vi "Tracking IOL.vi"(5 "Trajectory Cluster":T3, 6 "OCT Z PID Gains":cluster{"Kp":dbl, "Kd":dbl, "Ki":dbl}={"Kp"=0.0003, "Kd"=0.0001, "Ki"=0.01}, 7 "Eye Model Cluster":T2={"X Grid"=[], "Y Grid"=[], "Za_true Surf"=[], "Iris Center"=[], "Zp_true Surf"=[], "Pinv"=[[1.0, 0.0], [0.0, 1.0]], "za_true"=5.0, "za_work"=1.0, "zp_work"=-1.0, "zp_true"=-5.0}, 8 "error in":errorcluster, 9 "OCT Prev Posit":dbl, 10 "Resume Index":i32, 11 "FPGA VI Reference In":refnum<k20>) -> (0 "error out":errorcluster, 1 "OCT Last Posit":dbl, 2 "Leave Index":i32, 3 "FPGA VI Reference Out":refnum<k20>)   [LabVIEW 2016]
uses:
  Subsystems/Global Variables.vi
  <vilib>/Platform/TimedLoop/XDataNode/wakeup.ctl
  <vilib>/Platform/TimedLoop/XDataNode/XDNodeRunTimeDep.lvlib
  <vilib>/Platform/TimedLoop/XDataNode/nitl_modes.ctl
  <vilib>/Platform/TimedLoop/XDataNode/timing_clust.ctl
  <vilib>/platform/TimedLoop/XDataNode/XDataNode.xnode
  Library/KevinLibraryAll/labview/KevLib01.lvlib
  <vilib>/Analysis/Matrix/Datatypes/RealMatrix.ctl
  <vilib>/Analysis/Matrix/NI_Matrix.lvlib
panel:
  out "In Servo Loop":bool
  out "PC z Displacement":dbl
  out "Speed Schedule":dbl
  out "joint limits":dbl[][](array[numeric])=[[-10.0, 35.0], [-35.0, 35.0], [0.1, 10.0], [-40.0, 40.0]]
  out "Vac Extremum":dbl[](array[numeric])
  out "z Dist Thld":dbl[](array[numeric])
  out "z Rot Axis":dbl
  out "Deform Array":dbl[](array[numeric])=[1.0, 1.0, 1.0, 0.0, 0.0, 0.0, 0.0, 0.0, 0.0]
  out "Speed Override":u16(ring)=3 items=["4x", "3x", "2x", "1x", "0.5x", "0.2x", "0.1x", "PAUSE"]
  out "Loading Finished":bool
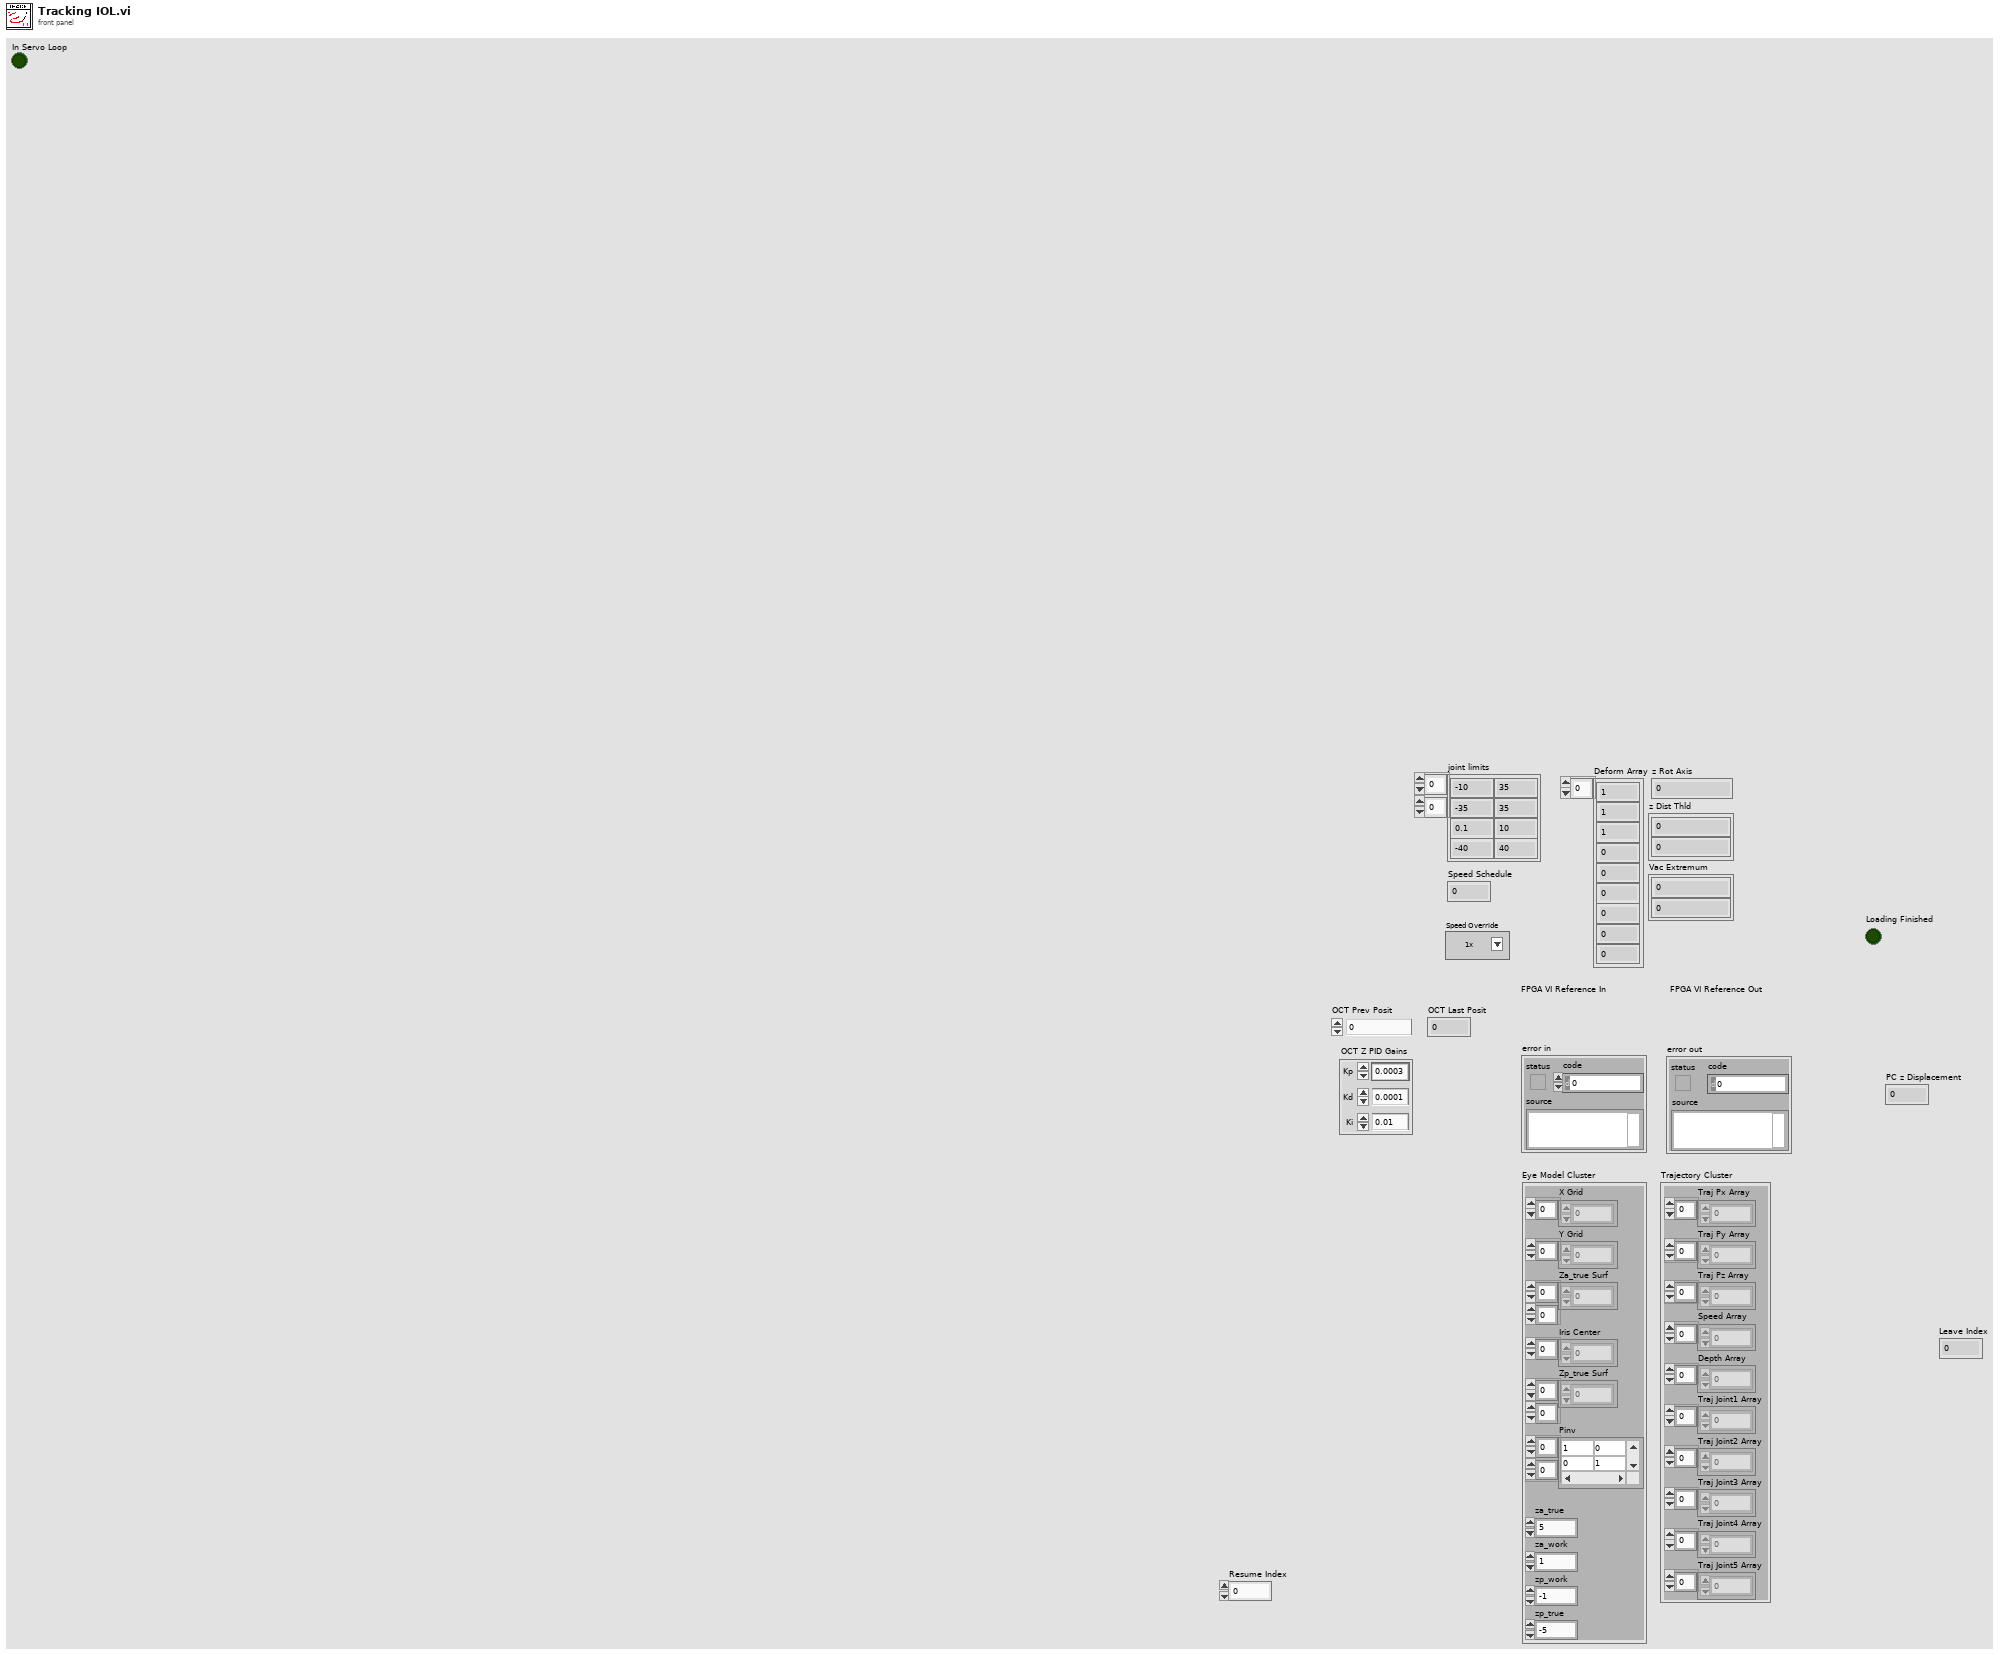
[diagram p1: front panel]
types:
  T1 = typedef "NI_Matrix.lvlib/RealMatrix.ctl" = dbl[][]
  T2 = cluster{"X Grid":dbl[], "Y Grid":dbl[], "Za_true Surf":dbl[][], "Iris Center":dbl[], "Zp_true Surf":dbl[][], "Pinv":T1, "za_true":dbl, "za_work":dbl, "zp_work":dbl, "zp_true":dbl}
  T3 = cluster{"Traj Px Array":dbl[], "Traj Py Array":dbl[], "Traj Pz Array":dbl[], "Speed Array":dbl[], "Depth Array":dbl[], "Traj Joint1 Array":dbl[], "Traj Joint2 Array":dbl[], "Traj Joint3 Array":dbl[], "Traj Joint4 Array":dbl[], "Traj Joint5 Array":dbl[]}
  T4 = typedef "XDNodeRunTimeDep.lvlib/timing_clust.ctl" = cluster{"Expected End [f-1]":u64, "Actual End [f-1]":u64, "Finished Late? [f-1]":bool, "Expected End [i-1]":u64, "Actual End [i-1]":u64, "Finished Late? [i-1]":bool, "Expected Start [i]":u64, "Actual Start [i]":u64, "Expected Start [f]":u64, "Actual Start [f]":u64, "Source Name":string, "Structure Name":string, "Period":i64, "Deadline":i64, "Offset":i64, "Start":i64, "Priority":i32, "Timeout":i32, "Mode":T5, "Wakeup Reason":T6, "Error":errorcluster, "Source Type":string, "Secondary Source Type":string, "Global End Time":u64, "Global Start Time":u64, "Frame Duration":u64, "Iteration Duration":u64, "Assigned CPU":i32, "I/O Scan Engine Mode":u32}
  T5 = typedef "XDNodeRunTimeDep.lvlib/nitl_modes.ctl" = enum32{"No Change", "Process missed periods, maintain original phase", "Discard missed periods, maintain original phase", "Process missed periods, ignore original phase", "Discard missed periods, ignore original phase"}
  T6 = typedef "XDNodeRunTimeDep.lvlib/wakeup.ctl" = enum32{"Normal", "Aborted", "Asynchronous wakeup", "Timing source error", "Timed loop error", "Timeout"}
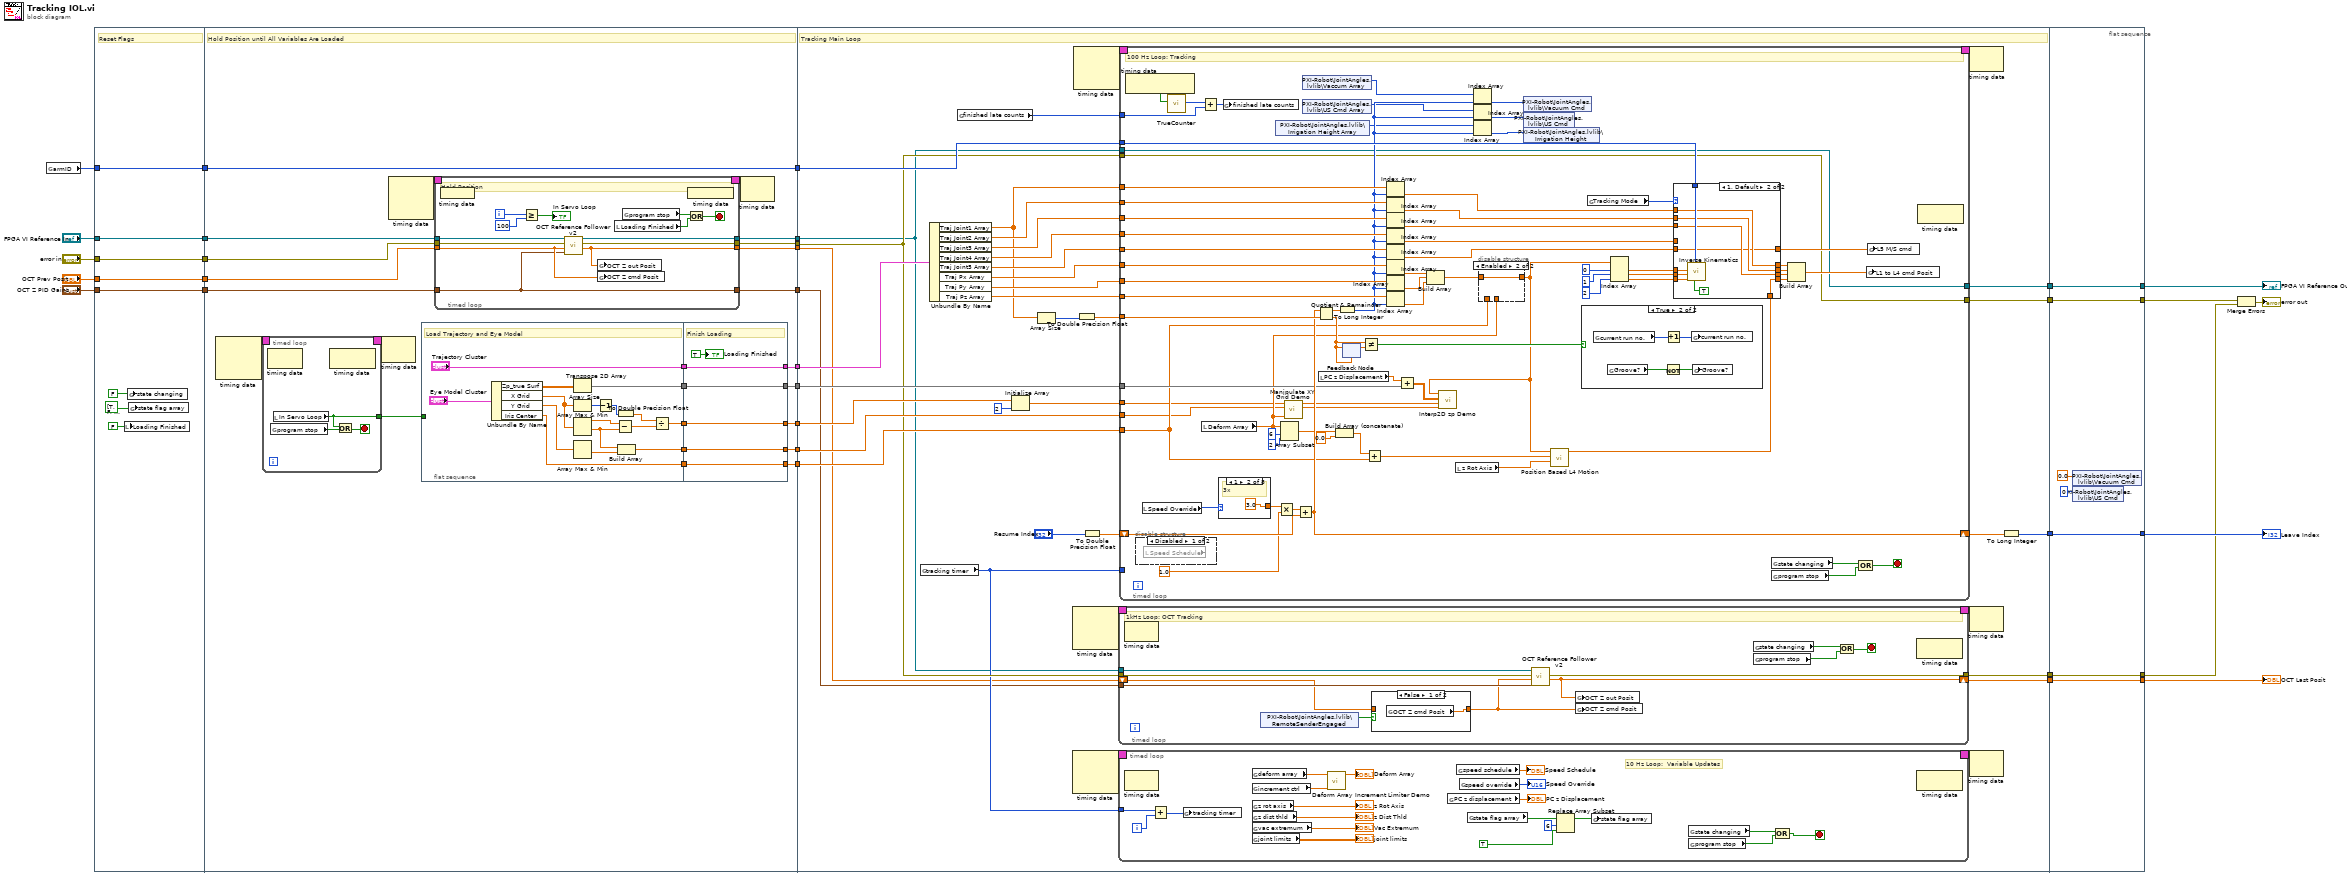
[diagram p0: block diagram]
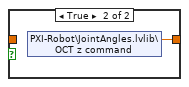
[diagram p2: hidden frame]
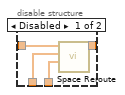
[diagram p5: hidden frame]
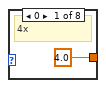
[diagram p6: hidden frame]
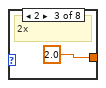
[diagram p7: hidden frame]
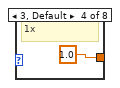
[diagram p8: hidden frame]
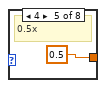
[diagram p9: hidden frame]
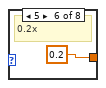
[diagram p10: hidden frame]
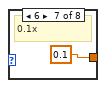
[diagram p11: hidden frame]
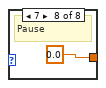
[diagram p12: hidden frame]
diagram:
  n1 = global read "Global Variables.vi" "armID"() -> (w13:i32)
  n2 = flat-sequence {
    tunnel: [w37] -> w31
    tunnel: "FPGA VI Reference In" -> [w37]
    tunnel: "error in" -> [w36]
    tunnel: [w36] -> w28
    tunnel: w13 -> [w35]
    tunnel: [w35] -> w15
    tunnel: [w33] -> w12
    tunnel: "OCT Prev Posit" -> [w33]
    tunnel: [w32] -> w10
    tunnel: "OCT Z PID Gains" -> [w32]
    tunnel: w31 -> [w50]
    tunnel: w28 -> [w49]
    tunnel: [w45] -> w27
    tunnel: [w63] -> w23
    tunnel: [w62] -> w22
    tunnel: [w61] -> w21
    tunnel: [w60] -> w19
    tunnel: [w59] -> w18
    tunnel: [w53] -> w17
    tunnel: w15 -> [w53]
    tunnel: [w46] -> w14
    tunnel: w12 -> [w48]
    tunnel: w10 -> [w47]
    tunnel: [w41] -> w8
    tunnel: [w40] -> w7
    tunnel: w27 -> [w125]
    tunnel: w23 -> [w139]
    tunnel: w22 -> [w131]
    tunnel: w21 -> [w140]
    tunnel: w19 -> [w132]
    tunnel: w18 -> [w133]
    tunnel: w17 -> [w128]
    tunnel: w14 -> [w122]
    tunnel: w8 -> [w121]
    tunnel: w7 -> [w120]
    tunnel: [w144] -> w5
    tunnel: [w143] -> w4
    tunnel: [w136] -> w3
    tunnel: [w124] -> w2
    tunnel: [w119] -> w1
    tunnel: [w304] -> w6
    tunnel: [w305] -> w16
    tunnel: [w306] -> w20
    tunnel: [w307] -> w24
    tunnel: [w308] -> w25
    tunnel: w5 -> [w308]
    tunnel: w4 -> [w307]
    tunnel: w3 -> [w306]
    tunnel: w2 -> [w305]
    tunnel: w1 -> [w304]
    frame #0 {
      # "Reset Flags"
      n3 = local write "Loading Finished"(FALSE ("Loading Finished")) -> ()
      n4 = global write "Global Variables.vi" "state changing"(FALSE ("state changing")) -> ()
      n5 = global write "Global Variables.vi" "state flag array"(bool[] [TRUE, FALSE, FALSE, FALSE, FALSE, FALSE, FALSE, FALSE, FALSE] ("state flag array")) -> ()
    }
    frame #1 {
      # "Hold Position until All Variables Are Loaded"
      n6 = node-c288() -> (w44:T4)  [unwired: 3 in]
      n7 = timed-loop {
        timing: w44 -> [_]
        timing-out: [_] -> w43
        tunnel: [w64] -> w42
        stop <- w66 stop-if-true
        n8 = node-c288() -> ()  [unwired: 1 in, 1 out]
        n9 = global read "Global Variables.vi" "program stop"() -> (w65:bool)
        n10 = local read "In Servo Loop"() -> (w64:bool)
        n11 = node-c288() -> ()  [unwired: 1 in, 1 out]
        n12 = Or(x=w64, y=w65) -> (x .or. y?=w66:bool)
      }
      n13 = node-c288(w43) -> ()  [unwired: 1 out]
      n14 = node-c288() -> (w52:T4)  [unwired: 3 in]
      n15 = flat-sequence {
        tunnel: [w90] -> w58
        tunnel: [w103] -> w57
        tunnel: [w102] -> w56
        tunnel: [w89] -> w55
        tunnel: ["Trajectory Cluster"] -> w54
        tunnel: w42 -> [_]
        tunnel: [w107] -> w61
        tunnel: [w108] -> w62
        tunnel: [w109] -> w63
        tunnel: w58 -> [w109]
        tunnel: w57 -> [w108]
        tunnel: w56 -> [w107]
        tunnel: w55 -> [w105]
        tunnel: [w105] -> w60
        tunnel: [w104] -> w59
        tunnel: w54 -> [w104]
        frame #0 {
          # "Load Trajectory and Eye Model"
          n16 = Unbundle By Name("Eye Model Cluster") -> ("Zp_true Surf"=w91:dbl[][], "X Grid"=w92:dbl[], "Y Grid"=w101:dbl[], "Iris Center"=w89:dbl[])
          n17 = Transpose 2D Array(2D array=w91) -> (transposed array=w90:dbl[][])
          n18 = Array Size(array=w92) -> (size(s)=w100:i32)
          n19 = Array Max & Min(array=w92) -> (max value=w98:dbl, min value=w99:dbl)  [unwired: 2 out]
          n20 = Array Max & Min(array=w101) -> (min value=w97:dbl)  [unwired: 3 out]
          n21 = Decrement(x=w100) -> (x-1=w95:i32)
          n22 = Subtract(x=w98, y=w99) -> (x-y=w94:dbl)
          n23 = To Double Precision Float(number=w95) -> (double precision float=w96:dbl)
          n24 = Build Array(w99, w97) -> (w102:dbl[])
          n25 = Divide(x=w96, y=w94) -> (x/y=w103:dbl)
        }
        frame #1 {
          # "Finish Loading"
          "Loading Finished" <- TRUE ("Loading Finished")
        }
      }
      n26 = timed-loop {
        timing: w52 -> [_]
        timing-out: [_] -> w51
        tunnel: [w74] -> w40
        tunnel: [w71] -> w46
        tunnel: [w75] -> w45
        tunnel: w50 -> [w77]
        tunnel: w49 -> [w76]
        tunnel: w47 -> [w72]
        tunnel: w48 -> [w73]
        tunnel: [w72] -> w41
        i -> [w80]
        stop <- w83 stop-if-true
        # "Hold Position"
        n27 = node-c288 ("Output Node")() -> ()  [unwired: 1 in]
        n28 = Greater Or Equal?(x=w80, y=100) -> (x >= y?=→"In Servo Loop":bool)
        n29 = call "OCT Reference Follower v2.vi"("OCT Z PID Gains"=w72, "OCT  Z cmd Posit [mm]"=w73, "error in"=w76, "FPGA VI Reference In"=w77) -> ("OCT  Z out Posit [mm]"=w74:dbl, "error out"=w75:errorcluster, "FPGA VI Reference Out"=w71:refnum<k20>)  [unwired: 5 in]
        n30 = global write "Global Variables.vi" "OCT Z out Posit"(w74) -> ()
        n31 = global write "Global Variables.vi" "OCT Z cmd Posit"(w73) -> ()
        n32 = local read "Loading Finished"() -> (w82:bool)
        n33 = global read "Global Variables.vi" "program stop"() -> (w81:bool)
        n34 = Or(x=w81, y=w82) -> (x .or. y?=w83:bool)
        n35 = node-c288() -> ()  [unwired: 1 out]
      }
      n36 = node-c288(w51) -> ()  [unwired: 1 out]
    }
    frame #2 {
      # "Tracking Main Loop"
      n37 = global read "Global Variables.vi" "tracking timer"() -> (w123:i32)
      n38 = Unbundle By Name(w133) -> ("Traj Joint1 Array"=w112:dbl[], "Traj Joint2 Array"=w118:dbl[], "Traj Joint3 Array"=w117:dbl[], "Traj Joint4 Array"=w116:dbl[], "Traj Joint5 Array"=w113:dbl[], "Traj Px Array"=w115:dbl[], "Traj Py Array"=w138:dbl[], "Traj Pz Array"=w134:dbl[])
      n39 = global read "Global Variables.vi" "finished late counts"() -> (w145:u16)
      n40 = Initialize Array(w131, 2 ("dimension size")) -> (w129:dbl[])
      n41 = Array Size(array=w112) -> (size(s)=w111:i32)
      n42 = node-c288() -> (w127:T4)  [unwired: 3 in]
      n43 = node-c288() -> (w142:T4)  [unwired: 3 in]
      n44 = node-c288() -> (w147:T4)  [unwired: 3 in]
      n45 = To Double Precision Float(number=w111) -> (double precision float=w114:dbl)
      n46 = To Double Precision Float(number="Resume Index") -> (double precision float=w135:dbl)
      n47 = timed-loop {
        timing: w127 -> [_]
        timing-out: [_] -> w126
        tunnel: w125 -> [w158]
        tunnel: [w157] -> w124
        tunnel: w122 -> [w156]
        tunnel: w121 -> [w155]
        shift-right: [w151] -> w119
        shift-left: w120 -> [w153]
        stop <- w148 stop-if-true
        # "1kHz Loop: OCT Tracking"
        n48 = node-c288() -> ()  [unwired: 1 in, 1 out]
        n49 = shared-variable "PXI-Robot\\JointAngles.lvlib\\RemoteSenderEngaged"() -> (w154:bool)  [unwired: 1 in, 1 out]
        n50 = case shown="False" w154 {
          tunnel: [w159 w160] -> w152
          tunnel: w153 -> [_ _]
          frame False {
            # "Hold Position if not Engaged"
            n51 = global read "Global Variables.vi" "OCT Z cmd Posit"() -> (w159:dbl)
          }
          frame True {
            n52 = shared-variable "PXI-Robot\\JointAngles.lvlib\\OCT z command"() -> (w160:dbl)  [unwired: 1 in, 1 out]
          }
        }
        n53 = call "OCT Reference Follower v2.vi"("OCT Z PID Gains"=w155, "OCT  Z cmd Posit [mm]"=w152, "error in"=w158, "FPGA VI Reference In"=w156) -> ("OCT  Z out Posit [mm]"=w151:dbl, "error out"=w157:errorcluster)  [unwired: 5 in, 1 out]
        n54 = global write "Global Variables.vi" "OCT Z out Posit"(w151) -> ()
        n55 = global write "Global Variables.vi" "OCT Z cmd Posit"(w152) -> ()
        n56 = global read "Global Variables.vi" "state changing"() -> (w150:bool)
        n57 = global read "Global Variables.vi" "program stop"() -> (w149:bool)
        n58 = Compound Arithmetic op=OR(w150, w149) -> (w148:bool)
        n59 = node-c288() -> ()  [unwired: 1 in, 1 out]
      }
      n60 = timed-loop {
        timing: w142 -> [_]
        timing-out: [_] -> w141
        tunnel: w123 -> [w171]
        i -> [w172]
        stop <- w165 stop-if-true
        # "10 Hz Loop:  Variable Updates"
        n61 = node-c288() -> ()  [unwired: 1 in, 1 out]
        n62 = Add(x=w171, y=w172) -> (x+y=w173:i32)
        n63 = global write "Global Variables.vi" "tracking timer"(w173) -> ()
        n64 = global read "Global Variables.vi" "deform array"() -> (w170:dbl[])
        n65 = global read "Global Variables.vi" "increment ctrl"() -> (w169:dbl[])
        n66 = global read "Global Variables.vi" "z rot axis"() -> (→"z Rot Axis":dbl)
        n67 = global read "Global Variables.vi" "z dist thld"() -> (→"z Dist Thld":dbl[])
        n68 = global read "Global Variables.vi" "vac extremum"() -> (→"Vac Extremum":dbl[])
        n69 = global read "Global Variables.vi" "joint limits"() -> (→"joint limits":dbl[][])
        n70 = call "Deform Array Increment Limiter Demo.vi"("Increment Array"=w169, "Defrom Ref"=w170) -> ("Deform Output"=→"Deform Array":dbl[])  [unwired: 9 in]
        n71 = global read "Global Variables.vi" "PC z displacement"() -> (→"PC z Displacement":dbl)
        n72 = global read "Global Variables.vi" "speed schedule"() -> (→"Speed Schedule":dbl)
        n73 = global read "Global Variables.vi" "speed override"() -> (→"Speed Override":u16)
        n74 = global read "Global Variables.vi" "state flag array"() -> (w176:bool[])
        n75 = Replace Array Subset(array=w176, new element=TRUE ("new element/subarray"), index=6) -> (w177:bool[])
        n76 = global write "Global Variables.vi" "state flag array"(w177) -> ()
        n77 = global read "Global Variables.vi" "state changing"() -> (w167:bool)
        n78 = global read "Global Variables.vi" "program stop"() -> (w166:bool)
        n79 = Compound Arithmetic op=OR(w167, w166) -> (w165:bool)
        n80 = node-c288() -> ()  [unwired: 1 in, 1 out]
      }
      n81 = timed-loop {
        timing: w147 -> [_]
        timing-out: [_] -> w146
        tunnel: w115 -> [w264]
        tunnel: w138 -> [w263]
        tunnel: w134 -> [w258]
        tunnel: w122 -> [w190]
        tunnel: w125 -> [w189]
        tunnel: [w190] -> w144
        tunnel: w145 -> [w259]
        tunnel: [w189] -> w143
        shift-right: [w245] -> w137
        shift-left: w135 -> [w248]
        tunnel: w139 -> [w241]
        tunnel: w129 -> [w238]
        tunnel: w140 -> [w237]
        tunnel: w114 -> [w247]
        tunnel: w132 -> [w240]
        tunnel: w123 -> [_]
        tunnel: w128 -> [w215]
        tunnel: w112 -> [w212]
        tunnel: w118 -> [w213]
        tunnel: w117 -> [w214]
        tunnel: w116 -> [w205]
        tunnel: w113 -> [w204]
        stop <- w198 stop-if-true
        # "100 Hz Loop: Tracking"
        n82 = node-c288() -> (w262:bool)  [unwired: 1 in]
        n83 = disable-structure shown="Disabled" {
          frame Disabled {
            n84 = local read "Speed Schedule"() -> ()  [unwired: 1 out]
          }
          frame Enabled {
          }
        }
        n85 = local read "Speed Override"() -> (w250:u16)
        n86 = call "TrueCounter.vi"("True?"=w262) -> ("True Count"=w260:u16)  [unwired: 10 in]
        n87 = Add(x=w260, y=w259) -> (x+y=w261:u16)
        n88 = local read "Deform Array"() -> (w239:dbl[])
        n89 = case shown="1" w250 {
          tunnel: [4.0 ("y") 3.0 ("y") 2.0 ("y") 1.0 ("y") 0.5 ("y") 0.2 ("y") 0.1 ("y") 0.0 ("y")] -> w249
          frame 0 {
            # "4x"
          }
          frame 1 {
            # "3x"
          }
          frame 2 {
            # "2x"
          }
          frame 3, Default {
            # "1x"
          }
          frame 4 {
            # "0.5x"
          }
          frame 5 {
            # "0.2x"
          }
          frame 6 {
            # "0.1x"
          }
          frame 7 {
            # "Pause"
          }
        }
        n90 = global write "Global Variables.vi" "finished late counts"(w261) -> ()
        n91 = shared-variable "PXI-Robot\\JointAngles.lvlib\\Irrigation Height Array"() -> (w196:i32[])  [unwired: 1 in, 1 out]
        n92 = Multiply(x=w249, y=1.0) -> (x*y=w251:dbl)
        n93 = Array Subset(array=w239, index=6, length=2) -> (w225:dbl[])
        n94 = call "Manipulate XY Grid Demo.vi"("Deform Array"=w239, "XY Grid min In"=w237, "XY Quant. Fact. In"=w238) -> ("XY Grid min Out"=w220:dbl[], "XY Quant. Fact. Out"=w221:dbl[])  [unwired: 7 in]
        n95 = Add(x=w251, y=w248) -> (x+y=w245:dbl)
        n96 = shared-variable "PXI-Robot\\JointAngles.lvlib\\Vaccum Array"() -> (w195:i32[])  [unwired: 1 in, 1 out]
        n97 = shared-variable "PXI-Robot\\JointAngles.lvlib\\US Cmd Array"() -> (w194:i32[])  [unwired: 1 in, 1 out]
        n98 = Quotient & Remainder(x=w245, y=w247) -> (x-y*floor(x/y)=w246:dbl, floor(x/y)=w242:dbl)
        n99 = local read "PC z Displacement"() -> (w228:dbl)
        n100 = Build Array (concatenate)(w225, 0.0) -> (w224:dbl[])
        n101 = To Long Integer(number=w246) -> (32bit integer=w197:i32)
        n102 = feedback-in #1(w242) -> ()
        n103 = feedback #1(w242) -> (w244:dbl)
        n104 = Not Equal?(x=w242, y=w244) -> (x != y?=w243:bool)
        n105 = Add(x=w224, y=w240) -> (x+y=w219:dbl[])
        n106 = Index Array(array=w212, index=w197) -> (element=w210:dbl)
        n107 = Index Array(array=w213, index=w197) -> (element=w209:dbl)
        n108 = Index Array(array=w214, index=w197) -> (element=w208:dbl)
        n109 = Index Array(array=w205, index=w197) -> (element=w203:dbl)
        n110 = Index Array(array=w204, index=w197) -> (element=w202:dbl)
        n111 = Index Array(array=w264, index=w197) -> (element=w254:dbl)
        n112 = Index Array(array=w263, index=w197) -> (element=w253:dbl)
        n113 = Index Array(array=w258, index=w197) -> (element=w252:dbl)
        n114 = Add(x=w228, y=w241) -> (x+y=w222:dbl[][])
        n115 = Build Array(w254, w253, w252) -> (w236:dbl[])
        n116 = local read "z Rot Axis"() -> (w218:dbl)
        n117 = Index Array(array=w195, index=w197) -> (element=w191:i32)
        n118 = Index Array(array=w194, index=w197) -> (element=w193:i32)
        n119 = Index Array(array=w196, index=w197) -> (element=w192:i32)
        n120 = disable-structure shown="Enabled" {
          disable-tunnel: w240 -> [w283 _]
          disable-tunnel: w239 -> [w282 _]
          disable-tunnel: w236 -> [w281 w284]
          disable-tunnel: [w280 w284] -> w217
          frame Disabled {
            n121 = call "Space Reroute.vi"("Deform Array"=w282, "Pivot Pt"=w283, "Nominal Traj Pt"=w281) -> ("Reroute Traj Pt"=w280:dbl[])  [unwired: 8 in]
          }
          frame Enabled {
          }
        }
        n122 = call "Interp2D zp Demo.vi"("XY Grid min"=w220, "XY Quantization Factor"=w221, "Zp array"=w222, "Tip Position"=w217) -> ()  [unwired: 7 in, 1 out]
        n123 = shared-variable "PXI-Robot\\JointAngles.lvlib\\Vacuum Cmd"(w191) -> ()  [unwired: 1 in, 1 out]
        n124 = shared-variable "PXI-Robot\\JointAngles.lvlib\\US Cmd"(w193) -> ()  [unwired: 1 in, 1 out]
        n125 = shared-variable "PXI-Robot\\JointAngles.lvlib\\Irrigation Height"(w192) -> ()  [unwired: 1 in, 1 out]
        n126 = call "Position Based L4 Motion.vi"("Assign z"=w218, "Iris Center"=w219, "Tip Position"=w217) -> ("L4 Motion [deg]"=w207:dbl)  [unwired: 8 in]
        n127 = case shown="True" w243 {
          frame False {
          }
          frame True {
            n128 = global read "Global Variables.vi" "current run no."() -> (w296:u8)
            n129 = global read "Global Variables.vi" "Groove?"() -> (w294:bool)
            n130 = Not(x=w294) -> (.not. x?=w293:bool)
            n131 = Increment(x=w296) -> (x+1=w295:u8)
            n132 = global write "Global Variables.vi" "current run no."(w295) -> ()
            n133 = global write "Global Variables.vi" "Groove?"(w293) -> ()
          }
        }
        n134 = global read "Global Variables.vi" "Tracking Mode"() -> (w211:u16)
        n135 = Index Array(array=w217, index #1=0 ("index"), index #2=1 ("index"), index #3=2 ("index")) -> (element #1=w235:dbl, element #2=w234:dbl, element #3=w233:dbl)
        n136 = case shown="1, Default" w211 {
          tunnel: w235 -> [_ w278]
          tunnel: w234 -> [_ w277]
          tunnel: w233 -> [_ w276]
          tunnel: [w269 w273] -> w232
          tunnel: [w268 w272] -> w231
          tunnel: [w267 w271] -> w230
          tunnel: w215 -> [_ w275]
          tunnel: w210 -> [w269 w273]
          tunnel: w209 -> [w268 w272]
          tunnel: w208 -> [w267 w271]
          tunnel: w207 -> [_ w274]
          tunnel: [w266 w274] -> w206
          tunnel: w203 -> [w266 _]
          tunnel: w202 -> [w265 w270]
          tunnel: [w265 w270] -> w201
          frame 0 {
          }
          frame 1, Default {
            n137 = call "Inverse Kinematics.vi"(6:TRUE ("isToolTipInsideEye"), "armID"=w275, "z"=w276, "y"=w277, "x"=w278) -> ()  [unwired: 3 in, 4 out]
          }
        }
        n138 = global read "Global Variables.vi" "state changing"() -> (w200:bool)
        n139 = global read "Global Variables.vi" "program stop"() -> (w199:bool)
        n140 = Build Array(w232, w231, w230, w206) -> (w229:dbl[])
        n141 = Compound Arithmetic op=OR(w200, w199) -> (w198:bool)
        n142 = global write "Global Variables.vi" "L1 to L4 cmd Posit"(w229) -> ()
        n143 = global write "Global Variables.vi" "L5 M/S cmd"(w201) -> ()
        n144 = node-c288() -> ()  [unwired: 1 in, 1 out]
      }
      n145 = node-c288(w126) -> ()  [unwired: 1 out]
      n146 = node-c288(w141) -> ()  [unwired: 1 out]
      n147 = node-c288(w146) -> ()  [unwired: 1 out]
      n148 = To Long Integer(number=w137) -> (32bit integer=w136:i32)
    }
    frame #3 {
      n149 = shared-variable "PXI-Robot\\JointAngles.lvlib\\Vacuum Cmd"(sgl 0.0 ("Vacuum Cmd")) -> ()  [unwired: 1 in, 1 out]
      n150 = shared-variable "PXI-Robot\\JointAngles.lvlib\\US Cmd"(0 ("US Cmd")) -> ()  [unwired: 1 in, 1 out]
    }
  }
  n151 = Merge Errors(w24, w16) -> (→"error out":errorcluster)
  "FPGA VI Reference Out" <- w25
  "Leave Index" <- w20
  "OCT Last Posit" <- w6
